vi "登陆程序.vi"() -> ()   [LabVIEW 2022 SP3]
panel:
  in  "身份类型:":string(combo)
  in  "退出":bool
  in  "登录":bool
  out "登陆结果":string
  in  "密码:":string
  in  "用户名:":string
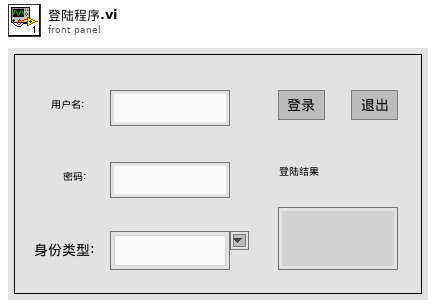
[diagram p1: front panel]
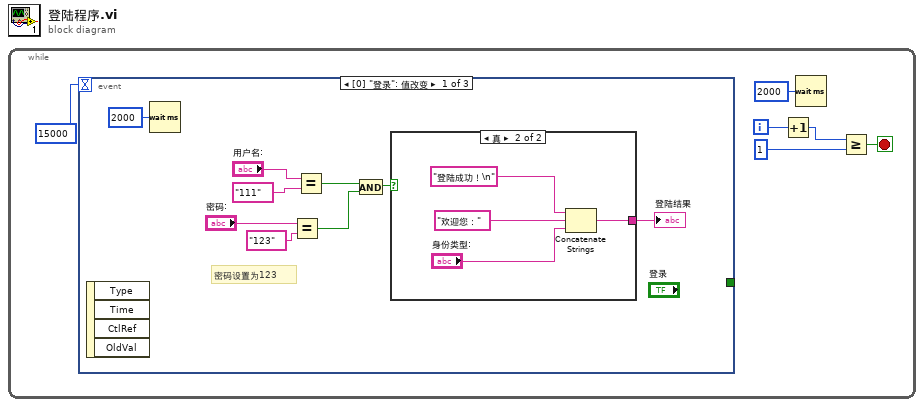
[diagram p0: block diagram]
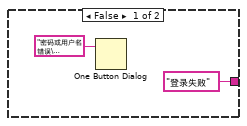
[diagram p2: hidden frame]
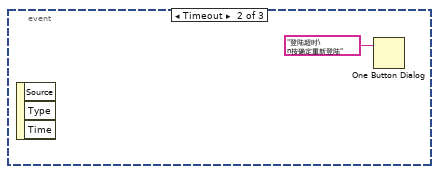
[diagram p3: hidden frame]
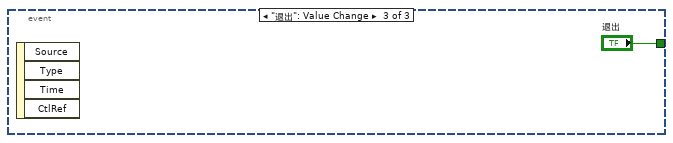
[diagram p4: hidden frame]
diagram:
  n1 = while {
    i -> [w2]
    stop <- w1 stop-if-true
    n2 = event shown="[0] \"登录\": 值改变" {
      selector: _ -> [_ _ _]
      dyn-events: _ -> [_ _ _]
      timeout: 15000 -> [_ _ _]
      tunnel: [_ _ "退出"] -> _
      event "登录": Value Change {
        # "密码设置为123"
        n3 = event-data() -> ()  [unwired: 5 out]
        n4 = Wait (ms)(milliseconds to wait=u32 2000 ("等待时间（毫秒）")) -> ()  [unwired: 1 out]
        n5 = Equal?(x="密码:", y="123") -> (x = y?=w11:bool)
        n6 = Equal?(x="用户名:", y="111") -> (x = y?=w12:bool)
        n7 = And(x=w12, y=w11) -> (x .and. y?=w13:bool)
        n8 = case shown="真" w13 {
          tunnel: ["登录失败" w21] -> w10
          frame False {
            n9 = One Button Dialog(message="密码或用户名错误\n请重新输入") -> ()  [unwired: 2 out]
          }
          frame True {
            n10 = Concatenate Strings("登陆成功！\n", "欢迎您：", "身份类型:") -> (w21:string)
          }
        }
        "登陆结果" <- w10
      }
      event Timeout {
        n11 = event-data() -> ()  [unwired: 4 out]
        n12 = One Button Dialog(message="登陆超时\n按确定重新登陆") -> ()  [unwired: 2 out]
      }
      event "退出": Value Change {
        n13 = event-data() -> ()  [unwired: 5 out]
      }
    }
    n14 = Increment ("加1")(x=w2) -> (x+1=w4:i32)
    n15 = Wait (ms)(milliseconds to wait=u32 2000 ("等待时间（毫秒）")) -> ()  [unwired: 1 out]
    n16 = Greater Or Equal?(x=w4, y=1) -> (x >= y?=w1:bool)
  }
